vi "channelcontrolsub.vi"(0 "TorqueSample":dbl, 1 "dt":dbl, 3 "Limit Number":dbl, 4 "Torque":bool, 5 "ControlPara":dbl[](array[numeric]), 7 "AngleSample":dbl, 8 "Angel":bool, 9 "syn-Error":dbl, 12 "Command":dbl, 16 "output range":cluster{"output high":dbl, "output low":dbl}, 17 "ChannelStatus":T1 items=["通道关", "位置通道", "加载通道"]) -> (19 "syn out":dbl, 20 "ControlOut":dbl, 22 "forward":dbl, 24 "diff syn out 2":dbl, 25 "PIDcontrol out":dbl, 27 "Commandout":dbl)   [LabVIEW 2020]
uses:
  Control 1.ctl
  <vilib>/Analysis/3filter.llb/Filter Passband Type.ctl
  <vilib>/addons/control/pid/pid.llb/PID (DBL).vi
  <vilib>/addons/control/pid/NI_PID_pid.lvlib
  <vilib>/ptbypt/NI_PtbyPt.lvlib
  <vilib>/Analysis/NI_AALBase.lvlib
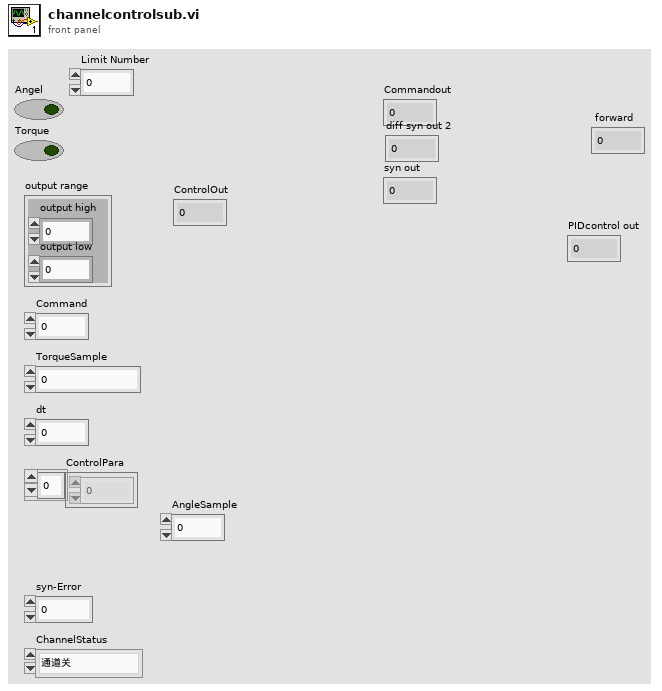
[diagram p1: front panel]
types:
  T1 = typedef "Control 1.ctl" = i32
  T2 = typedef "NI_AALBase.lvlib/Filter Passband Type.ctl" = enum32{"Lowpass", "Highpass", "Bandpass", "Bandstop"}
  T3 = cluster{"Numeric":dbl, "Numeric":dbl, "Numeric":dbl}
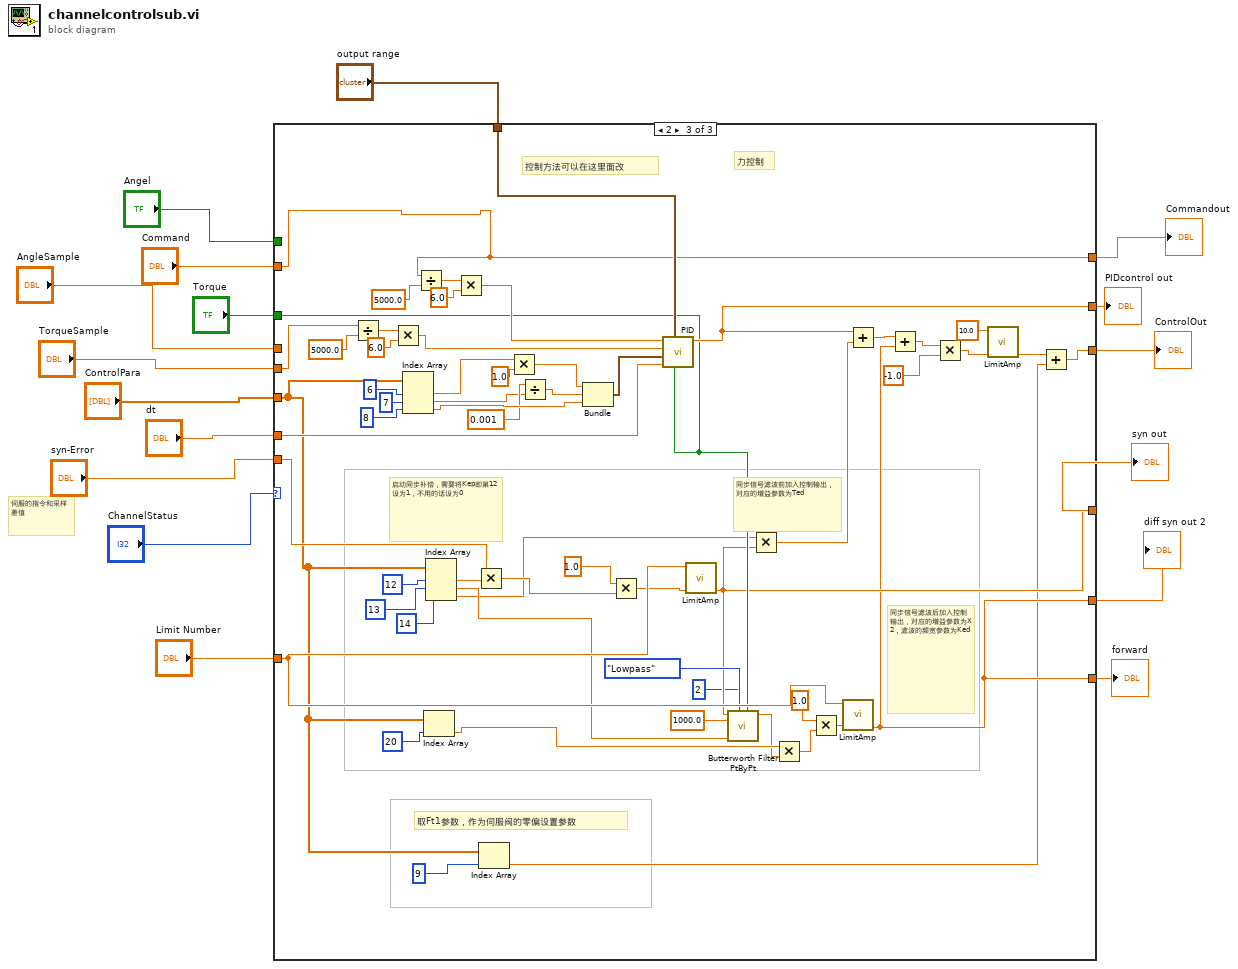
[diagram p0: block diagram]
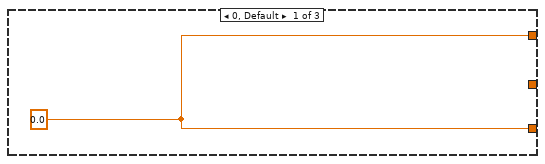
[diagram p2: hidden frame]
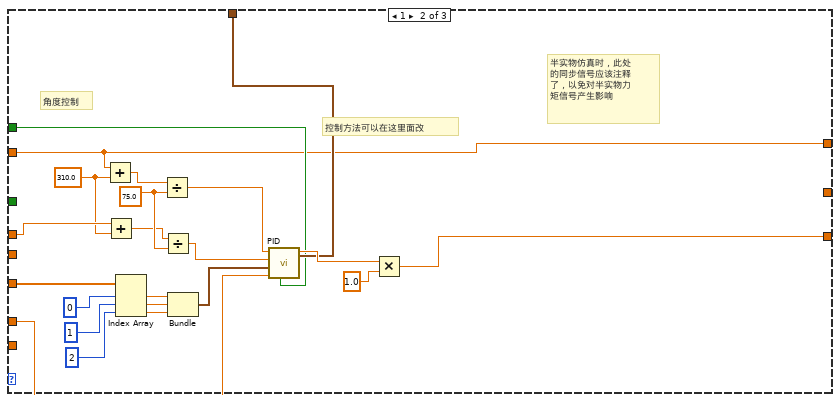
[diagram p3: hidden frame]
diagram:
  # "伺服的指令和采样差值"
  n1 = case shown="2" "ChannelStatus" {
    tunnel: "dt" -> [_ w31 w67]
    tunnel: "output range" -> [_ w30 w98]
    tunnel: "Command" -> [_ w24 w66]
    tunnel: "ControlPara" -> [_ w37 w47]
    tunnel: [w18 w28 w43] -> w16
    tunnel: "TorqueSample" -> [_ _ w83]
    tunnel: "syn-Error" -> [_ _ w48]
    tunnel: "AngleSample" -> [_ w23 _]
    tunnel: "Angel" -> [_ w27 _]
    tunnel: "Torque" -> [_ _ w62]
    tunnel: [w18 w24 w66] -> w7
    tunnel: [_ _ w77] -> w6
    tunnel: "Limit Number" -> [_ _ w74]
    tunnel: [_ _ w56] -> w2
    tunnel: [_ _ w52] -> w1
    tunnel: [_ _ w52] -> w4
    frame 0, Default {
      w18 = 0.0 ("output")
    }
    frame 1 {
      w21 = 75.0
      w22 = 310.0
      # "半实物仿真时，此处\n的同步信号应该注释\n了，以免对半实物力\n矩信号产生影响"
      # "控制方法可以在这里面改"
      # "角度控制"
      n2 = Add(x=w24, y=w22) -> (x+y=w26:dbl)
      n3 = Add(x=w23, y=w22) -> (x+y=w20:dbl)
      n4 = Index Array(array=w37, index #1=0 ("index"), index #2=1 ("index"), index #3=2 ("index")) -> (element #1=w35:dbl, element #2=w29:dbl, element #3=w34:dbl)
      n5 = Divide(x=w26, y=w21) -> (x/y=w25:dbl)
      n6 = Divide(x=w20, y=w21) -> (x/y=w19:dbl)
      n7 = Bundle("Numeric"=w35, "Numeric"=w29, "Numeric"=w34) -> (w32:T3)  [unwired: 1 in]
      n8 = call-poly <vilib>:"PID.vi"("reinitialize? (F)"=w27, "output range"=w30, "dt (s)"=w31, "PID gains"=w32, "process variable"=w19, "setpoint"=w25) -> ("output"=w33:dbl)  [unwired: 4 in, 1 out]
      n9 = Multiply(x=w33, y=1.0) -> (x*y=w28:dbl)
    }
    frame 2 {
      # "同步信号滤波前加入控制输出，对应的增益参数为Ted"
      # "同步信号滤波后加入控制输出，对应的增益参数为X2，滤波的频宽参数为Ked"
      # "取Ft1参数，作为伺服阀的零偏设置参数"
      # "启动同步补偿，需要将Kep即第12设为1，不用的话设为0"
      # "力控制"
      # "控制方法可以在这里面改"
      n10 = Divide(x=w83, y=5000.0) -> (x/y=w87:dbl)
      n11 = Multiply(x=w87, y=6.0) -> (x*y=w86:dbl)
      n12 = Index Array(array=w47, index #1=6 ("index"), index #2=7 ("index"), index #3=8 ("index")) -> (element #1=w70:dbl, element #2=w68:dbl, element #3=w85:dbl)
      n13 = Divide(x=w66, y=5000.0) -> (x/y=w91:dbl)
      n14 = Index Array(array=w47, index=20) -> (element=w65:dbl)
      n15 = Index Array(array=w47, index #1=12 ("index"), index #2=13 ("index"), index #3=14 ("索引")) -> (element #1=w64:dbl, element #2=w60:dbl, element #3=w50:dbl)
      n16 = Multiply(x=w91, y=6.0) -> (x*y=w90:dbl)
      n17 = Multiply(x=w48, y=w64) -> (x*y=w75:dbl)
      n18 = Index Array(array=w47, index=9 ("索引")) -> (element=w45:dbl)
      n19 = Multiply(x=w70, y=1.0) -> (x*y=w81:dbl)
      n20 = Divide(x=0.001 ("y"), y=w68) -> (x/y=w80:dbl)
      n21 = Bundle(w81, w80, "Numeric"=w85) -> (w94:cluster{dbl, dbl, "Numeric":dbl})  [unwired: 1 in]
      n22 = Multiply(x=1.0 ("y"), y=w75) -> (x*y=w41:dbl)
      n23 = call-poly <vilib>:"PID.vi"("reinitialize? (F)"=w62, "output range"=w98, "dt (s)"=w67, "PID gains"=w94, "process variable"=w86, "setpoint"=w90) -> ("output"=w77:dbl)  [unwired: 4 in, 1 out]
      n24 = call "LimitAmp.vi"("data in"=w41, "limit"=w74) -> ("data out"=w56:dbl)  [unwired: 9 in]
      n25 = call <vilib>:"Butterworth Filter PtByPt.vi"("initialize"=w62, "order"=2, "filter type"=Filter_Passband_Type."Lowpass", "low cutoff freq: fl"=w60, "sampling freq: fs"=1000.0, "x"=w56) -> ("Filtered x"=w49:dbl)  [unwired: 3 in, 1 out]
      n26 = Multiply(x=w50, y=w56) -> (x*y=w55:dbl)
      n27 = Multiply(x=w65, y=w49) -> (x*y=w57:dbl)
      n28 = Multiply(x=1.0 ("y"), y=w57) -> (x*y=w58:dbl)
      n29 = call "LimitAmp.vi"("data in"=w58, "limit"=w74) -> ("data out"=w52:dbl)  [unwired: 9 in]
      n30 = Add(x=w77, y=w55) -> (x+y=w73:dbl)
      n31 = Add(x=w73, y=w52) -> (x+y=w72:dbl)
      n32 = Multiply(x=w72, y=-1.0) -> (x*y=w54:dbl)
      n33 = call "LimitAmp.vi"("data in"=w54, "limit"=10.0) -> ("data out"=w44:dbl)  [unwired: 9 in]
      n34 = Add(x=w44, y=w45) -> (x+y=w43:dbl)
    }
  }
  "ControlOut" <- w16
  "Commandout" <- w7
  "syn out" <- w2
  "PIDcontrol out" <- w6
  "forward" <- w1
  "diff syn out 2" <- w4
